vi "OOI Input Dialog.vi"(0 "Enable":bool=TRUE, 5 "error in (no error)":errorcluster) -> (9 "Additional Information":string, 11 "Normal relevance":bool, 12 "High relevance":bool, 15 "Coral Reef":bool, 16 "Ship Wreck":bool, 17 "Artifact":bool, 18 "OK":bool, 19 "error out":errorcluster)   [LabVIEW 2012]
doc: "Displays a standard dialog box that prompts users to enter information, such as a user name and password.\n--------------------\n\nThis Express VI is configured as follows:\n\nMessage to Display to the User:Insert details of the Object Of Interest\nThe inputs are: \nCheckbox: Artifact\nCheckbox: Ship Wreck\nCheckbox: Coral Reef\nCheckbox: Interesting geology\nCheckbox: Interesting biology\nCheckbox: High relevance\nCheckbox: Normal relevance\nCheckbox: Low relevance\nText Entry Box: Additional Information"
panel:
  out "String 3":string="Insert details of the Object Of Interest" caption="String"
  out "String 2":string="Insert details of the Object Of Interest" caption="String"
  in  "ADDITIONAL NOTES":string caption="Additional Information"
  in  "Normal relevance":bool
  in  "High relevance":bool
  in  "Coral Reef":bool
  in  "Ship Wreck":bool
  in  "Artifact":bool
  out "String":string="Insert details of the Object Of Interest"
  in  "Cancel":bool
  in  "OK2":bool
  in  "OK1":bool
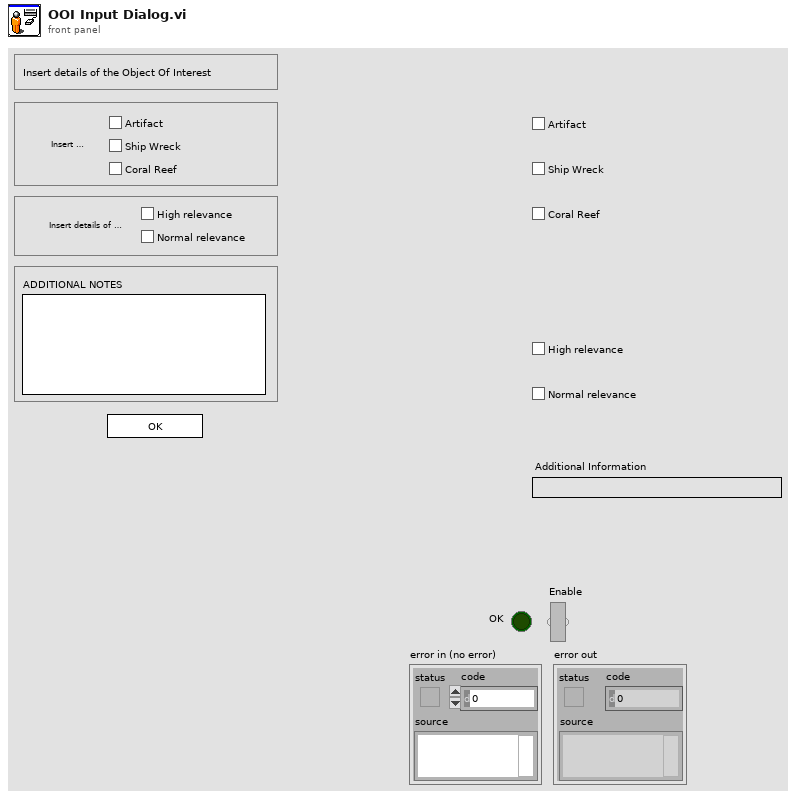
[diagram p1: front panel]
types:
  T1 = cluster{"Input Name":string, "Input Data Type":i32}[]
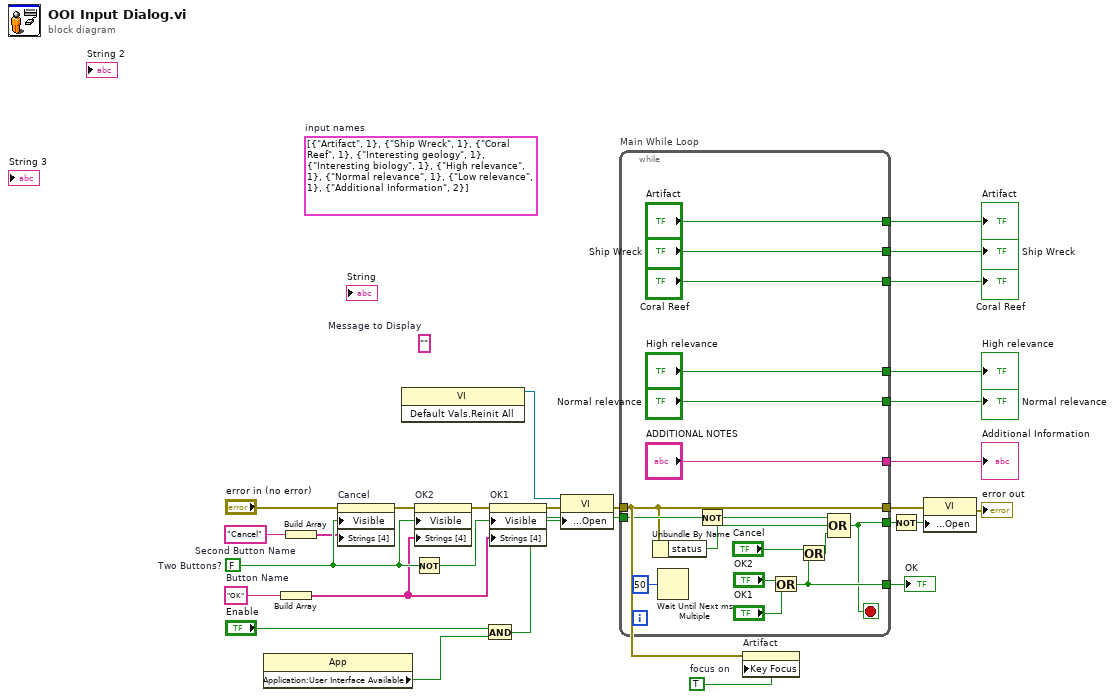
[diagram p0: block diagram]
diagram:
  w6 = TRUE  # focus on
  (unwired) T1 [{"Input Name"="Artifact", "Input Data Type"=1}, {"Input Name"="Ship Wreck", "Input Data Type"=1}, {"Input Name"="Coral Reef", "Input Data Type"=1}, {"Input Name"="Interesting geology", "Input Data Type"=1}, {"Input Name"="Interesting biology", "Input Data Type"=1}, {"Input Name"="High relevance", "Input Data Type"=1}, {"Input Name"="Normal relevance", "Input Data Type"=1}, {"Input Name"="Low relevance", "Input Data Type"=1}, {"Input Name"="Additional Information", "Input Data Type"=2}]  # input names
  w19 = "Cancel"  # Second Button Name
  w17 = "OK"  # Button Name
  (unwired) ""  # Message to Display
  w27 = FALSE  # Two Buttons?
  n1 = property class="App"() -> ("Application:User Interface Available"=w9:bool)  [unwired: 2 in, 2 out]
  n2 = Build Array(w17) -> (w18:string[])
  n3 = Build Array(w19) -> (w20:string[])
  n4 = property on="Cancel" class="Bool"(error in="error in (no error)", "Visible"=w27, "Strings [4]"=w20) -> (error out=w24:errorcluster)  [unwired: 1 in, 1 out]
  n5 = invoke class="VI" method="Default Vals.Reinit All"() -> (reference out=w8:refnum<vi>)  [unwired: 3 in, 2 out]
  n6 = Not(x=w27) -> (.not. x?=w25:bool)
  n7 = property on="OK2" class="Bool"(error in=w24, "Visible"=w27, "Strings [4]"=w18) -> (error out=w23:errorcluster)  [unwired: 1 in, 1 out]
  n8 = And(x="Enable", y=w9) -> (x .and. y?=w10:bool)
  n9 = property on="OK1" class="Bool"(error in=w23, "Visible"=w25, "Strings [4]"=w18) -> (error out=w16:errorcluster)  [unwired: 1 in, 1 out]
  n10 = property class="VI"(reference=w8, error in=w16, "Front Panel Window:Open"=w10) -> (error out=w15:errorcluster)  [unwired: 1 out]
  n11 = while "Main While Loop" {
    tunnel: [w41] -> w26
    tunnel: w10 -> [w39]
    tunnel: [w37] -> w21
    tunnel: w15 -> [w36]
    tunnel: [w36] -> w13
    tunnel: ["Artifact"] -> w7
    tunnel: ["Ship Wreck"] -> w5
    tunnel: ["Coral Reef"] -> w4
    tunnel: ["High relevance"] -> w3
    tunnel: ["Normal relevance"] -> w2
    tunnel: ["ADDITIONAL NOTES"] -> w1
    stop <- w37 stop-if-true
    n12 = Unbundle By Name(w36) -> ("status"=w34:bool)
    n13 = Wait Until Next ms Multiple(millisecond multiple=u32 50) -> ()  [unwired: 1 out]
    n14 = Not(x=w39) -> (.not. x?=w38:bool)
    n15 = Or(x="OK2", y="OK1") -> (x .or. y?=w41:bool)
    n16 = Or(x="Cancel", y=w41) -> (x .or. y?=w35:bool)
    n17 = Compound Arithmetic op=OR(w38, w34, w35) -> (w37:bool)
  }
  "OK" <- w26
  "Artifact" <- w7
  "Ship Wreck" <- w5
  "Coral Reef" <- w4
  "High relevance" <- w3
  "Normal relevance" <- w2
  "Additional Information" <- w1
  n18 = property on="Artifact" class="Bool (strict)"(error in=w15, "Key Focus"=w6) -> ()  [unwired: 1 in, 2 out]
  n19 = Not(x=w21) -> (.not. x?=w22:bool)
  n20 = property class="VI"(error in=w13, "Front Panel Window:Open"=w22) -> (error out=→"error out":errorcluster)  [unwired: 1 in, 1 out]
